vi "DRV.vi"(0 "System no.":i32=1 min=1 max=4 step=1, 2 "Strut to command":string, 3 "Mode":i32=1, 5 "error in":errorcluster) -> (19 "error out":errorcluster)   [LabVIEW 2020]
doc: "A spindle revolution of one single strut is performed while monitoring the motor current. For system maintenance purposes. User DRR?.vi or DRR? and display data.vi to read values back.\n\nC-887, F-206: Only for GCS syntax version = GCS 2.0 or higher (check with CSV?.vi. If CSV?.vi is not supported, syntax version is GCS 1.0). Requires command level 1 (CCL). Strut to command can be 1 to 6. Mode can be 1 (forward spindle rotation) or -1 (backward rotation) \n\nC-887, M-8X0: Only supported if controller is based on C-842.80 or GCS syntax version = GCS 2.0 or higher (check with CSV?.vi. If CSV?.vi is not supported, syntax version is GCS 1.0). For GCS 2.0, requires command level 1 (CCL). Strut to command can be 1 to 6. Mode can be 1 (forward spindle rotation) or -1 (backward rotation)"
panel:
  # "A spindle revolution of one single strut is performed while \nmonitoring the motor current. For system maintenance purposes.\nUser \"DRR?.vi\" or \"DRR? and display data.vi\" to read values back."
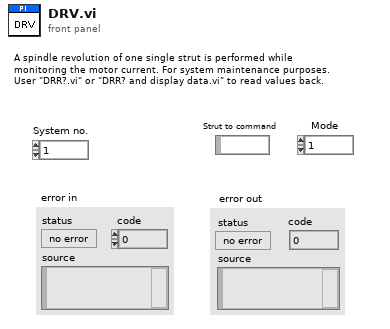
[diagram p1: front panel]
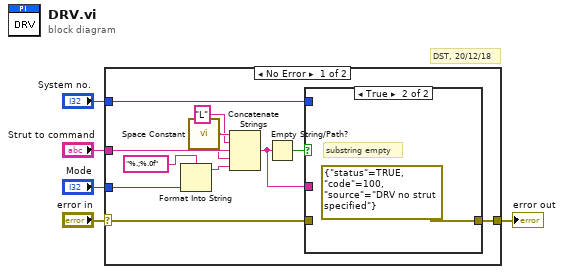
[diagram p0: block diagram]
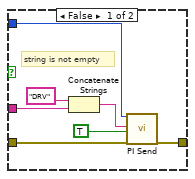
[diagram p2: hidden frame]
diagram:
  # "DST, 20/12/18"
  n1 = case shown="No Error" "error in" {
    selector: "error in" -> [w8 w25]
    tunnel: [w16 w25] -> w5
    tunnel: "System no." -> [w15 _]
    tunnel: "Strut to command" -> [w11 _]
    tunnel: "Mode" -> [w12 _]
    frame No Error {
      n2 = Format Into String(format string="%.;%.0f" ("Format String"), w12) -> (resulting string=w14:string)  [unwired: 2 in, 1 out]
      n3 = call <vilib>:"Space Constant.vi"() -> ("String"=w10:string)
      n4 = Concatenate Strings(w10, "L" ("string"), w11, w10, w14) -> (w7:string)
      n5 = Empty String/Path?(string/path=w7) -> (empty?=w6:bool)
      n6 = case shown="True" w6 {
        tunnel: w7 -> [w22 _]
        tunnel: [w18 errorcluster {"status"=TRUE, "code"=100, "source"="DRV no strut specified"} ("error out")] -> w16
        tunnel: w8 -> [w19 _]
        tunnel: w15 -> [w17 _]
        frame False {
          # "string is not empty"
          n7 = Concatenate Strings("DRV", w22) -> (w20:string)
          n8 = call "PI Send.vi"("System no."=w17, "String to send"=w20, "Attach termination char.?"=TRUE ("Attach Linefeed?"), "error in"=w19) -> ("error out"=w18:errorcluster)  [unwired: 2 in, 13 out]
        }
        frame True {
          # "substring empty"
        }
      }
    }
    frame Error {
    }
  }
  "error out" <- w5
